vi "s3path.set.vi"(8 "error in (no error)":errorcluster, 10 "s3path":string, 11 "s3path in":refnum<class "s3path.lvclass">) -> (0 "error out":errorcluster, 3 "s3path out":refnum<class "s3path.lvclass">)   [LabVIEW 2020, in "nominal types.lvlib" / "timestampManifest.lvlib" / "s3path.lvclass"]
uses:
  s3path.lvclass
  s3path.lvclass/s3path.ctl
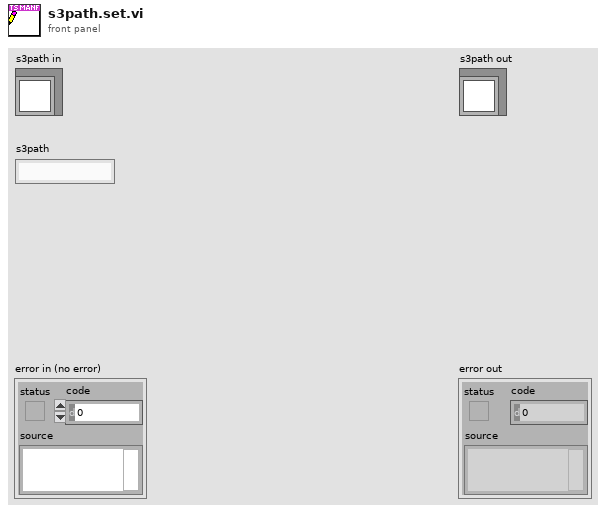
[diagram p1: front panel]
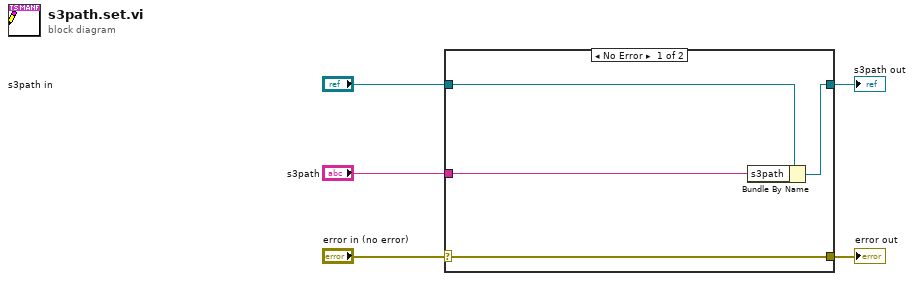
[diagram p0: block diagram]
diagram:
  n1 = case shown="No Error" "error in (no error)" {
    selector: "error in (no error)" -> [w9 w10]
    tunnel: [w9 w10] -> w4
    tunnel: [w7 w11] -> w2
    tunnel: "s3path in" -> [w8 w11]
    tunnel: "s3path" -> [w6 _]
    frame No Error {
      n2 = Bundle By Name(cluster=w8, "s3path"=w6) -> (w7:refnum<class "s3path.lvclass">)
    }
    frame Error {
    }
  }
  "error out" <- w4
  "s3path out" <- w2
